vi "Save config.vi"(8 "error in (no error)":errorcluster, 10 "Mono config":T1={"VISA resource "="", "nm/min"=100.0}, 11 "Lock-in config":T2) -> (0 "error out":errorcluster)   [LabVIEW 2020]
uses:
  controls/Lock-in config.ctl
  controls/Mono config.ctl
  <vilib>/Utility/config.llb/Write Key (String).vi
  <vilib>/Utility/config.llb/Write Key (Double).vi
  <vilib>/Utility/config.llb/NI_LVConfig.lvlib
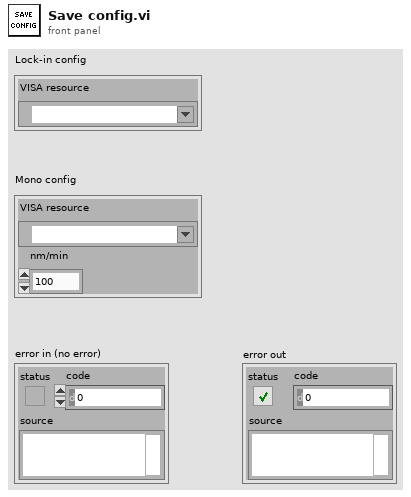
[diagram p1: front panel]
types:
  T1 = typedef "Mono config.ctl" = cluster{"VISA resource ":refnum<visa-resource-name>, "nm/min":dbl}
  T2 = typedef "Lock-in config.ctl" = cluster{"VISA resource ":refnum<visa-resource-name>}
  T3 = typedef "NI_LVConfig.lvlib/Config Data RefNum.ctl" = refnum<k1>
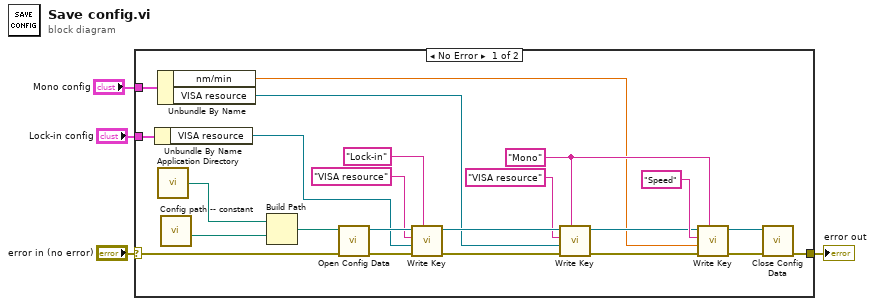
[diagram p0: block diagram]
diagram:
  n1 = case shown="No Error" "error in (no error)" {
    selector: "error in (no error)" -> [w25 w28]
    tunnel: [w24 w28] -> w3
    tunnel: "Lock-in config" -> [w19 _]
    tunnel: "Mono config" -> [w14 _]
    frame No Error {
      w11 = "Mono" ("section")
      n2 = Unbundle By Name(w19) -> ("VISA resource"=w18:refnum<visa-resource-name>)
      n3 = Unbundle By Name(w14) -> ("nm/min"=w8:dbl, "VISA resource"=w13:refnum<visa-resource-name>)
      n4 = call <vilib>:"Application Directory.vi"() -> ("Application Directory"=w27:path)
      n5 = call "Config path -- constant.vi"() -> ("name or relative path"=w5:path)  [unwired: 11 in]
      n6 = Build Path(base path=w27, name or relative path=w5) -> (appended path=w26:path)
      n7 = call <vilib>:"Open Config Data.vi"("error in (no error)"=w25, "configuration file path"=w26) -> ("error out"=w22:errorcluster, "refnum"=w21:T3)  [unwired: 7 in, 1 out]
      n8 = call-poly <vilib>:"Write Key.vi"("section"="Lock-in", "error in (no error)"=w22, "value"=w18, "key"="VISA resource", "refnum"=w21) -> ("error out"=w17:errorcluster, "refnum out"=w16:T3)  [unwired: 4 in, 1 out]
      n9 = call-poly <vilib>:"Write Key.vi"("section"=w11, "error in (no error)"=w17, "value"=w13, "key"="VISA resource", "refnum"=w16) -> ("error out"=w12:errorcluster, "refnum out"=w9:T3)  [unwired: 4 in, 1 out]
      n10 = call-poly <vilib>:"Write Key.vi"("section"=w11, "error in (no error)"=w12, "value"=w8, "key"="Speed", "refnum"=w9) -> ("error out"=w7:errorcluster, "refnum out"=w6:T3)  [unwired: 4 in, 1 out]
      n11 = call <vilib>:"Close Config Data.vi"("error in (no error)"=w7, "refnum"=w6) -> ("error out"=w24:errorcluster)  [unwired: 8 in, 1 out]
    }
    frame Error {
    }
  }
  "error out" <- w3
